vi "N6705B_Convert_dlog_to_csv.vi"(10 "File Name Out":string, 11 "VISA Refnum in":refnum<visa-resource-name>) -> ()   [LabVIEW 2015]
uses:
  <instrlib>/Agilent N6700 Series/Agilent N6700 Series.lvlib
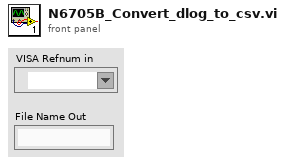
[diagram p1: front panel]
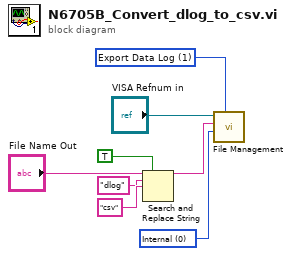
[diagram p0: block diagram]
diagram:
  w3 = 1 items=["Delete File", "Export Data Log"] ("Operation (1: Export Data Log)")
  w2 = 0 items=["Internal", "External"] ("File Location (0: Internal)")
  n1 = Search and Replace String(replace all?=TRUE ("replace all? (F)"), input string="File Name Out", search string="dlog", replace string="csv" ("replace string (\"\")")) -> (result string=w8:string)  [unwired: 4 in, 3 out]
  n2 = call <instrlib>:"File Management.vi"("Operation (1: Export Data Log)"=w3, "File Location (0: Internal)"=w2, "File Path"=w8, "VISA resource name"="VISA Refnum in") -> ()  [unwired: 6 in, 2 out]
